vi "RoperGasMeter.vi"() -> ()   [LabVIEW 2012]
uses:
  <vilib>/DAQmx/read.llb/DAQmx Read (Analog 1D DBL NChan 1Samp).vi
  <vilib>/DAQmx/miscellaneous.llb/DAQmx Fill In Error Info.vi
panel:
  out "Meter Flow":string
  out "NG":bool
  out "LP":bool
  out "Meter 6 Present":bool
  out "Meter 5 Present":bool
  out "Meter 4 Present":bool
  out "Meter 3 Present":bool
  out "Meter 2 Present":bool
  out "Meter 1 Present":bool
  out "Meter Type 6":string
  out "Meter Type 2":string
  out "Meter Type 4":string
  out "Meter Type 5":string
  out "Meter Type 3":string
  out "Meter Type 1":string
  out "Meter 6 Size":dbl
  out "Meter 5 Size":dbl
  out "Meter 4 Size":dbl
  out "Meter 3 Size":dbl
  out "Meter 2 Size":dbl
  out "Meter 1 Size":dbl
  out "ANSI Placeholder":dbl
  out "Start Time ANSI":dbl
  in  "Start ANSI":bool
  out "ANSI 5 Minute Average (BTU/hr)":dbl format="%#_5g"
  out "30 Second Average (BTU/hr)":dbl format="%#_5g"
  out "15 Second Average (BTU/hr)":dbl format="%#_5g"
  out "Reference6":dbl
  out "Reference5":dbl
  out "Reference4":dbl
  out "Reference3":dbl
  out "Reference2":dbl
  out "Reference1":dbl
  out "Time":dbl
  out "Num Record":dbl
  in  "HeatingValueLP":dbl=2450.0 min=2400.0 max=2600.0 step=5.0
  out "Output 6":dbl min=0.0 max=5.0 step=0.01
  out "Output 5":dbl min=0.0 max=5.0 step=0.01
  out "Output 4":dbl min=0.0 max=5.0 step=0.01
  out "Output 3":dbl min=0.0 max=5.0 step=0.01
  out "Output 2":dbl min=0.0 max=5.0 step=0.01
  out "Output 1":dbl min=0.0 max=5.0 step=0.01
  out "Signal":bool
  in  "Record":bool
  out "File Path":path
  out "CF/HR":dbl format="%#_2g"
  out "HV":dbl
  in  "HeatingValueNG":dbl=1000.0 min=950.0 max=1150.0 step=1.0
  out "Meter ID":dbl
  out "Gas":string
  out "DisplayChart":cluster{"Flow Rate":dbl}(graph)
  out "Flow Rate":dbl format="%#_5g"
  # "Instant Flow Rate (BTU/hr)"
  # "Dry Heating Value"
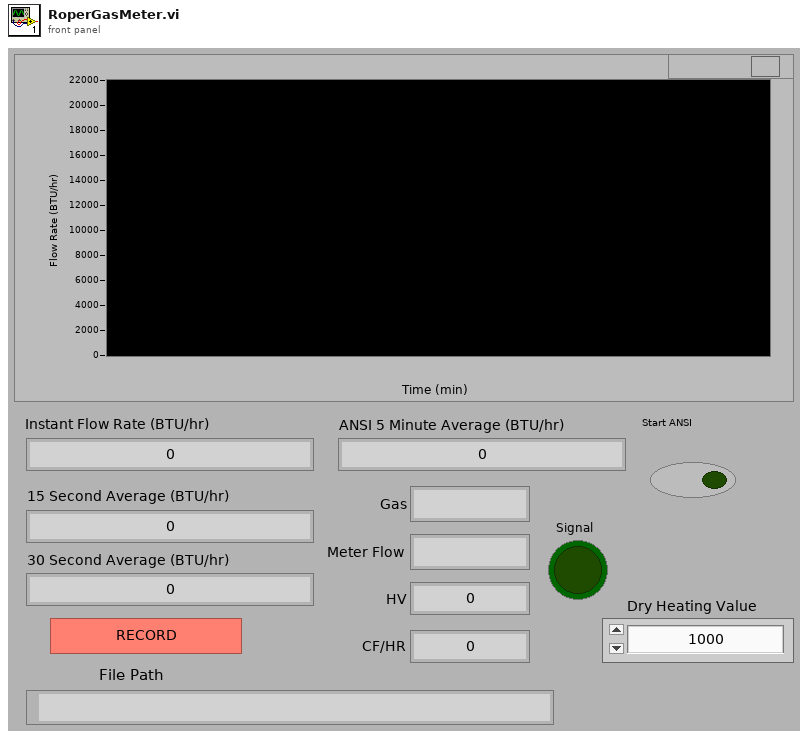
[diagram p1: front panel]
types:
  T1 = enum16{"open", "replace", "create", "open or create", "replace or create", "replace or create with confirmation"}
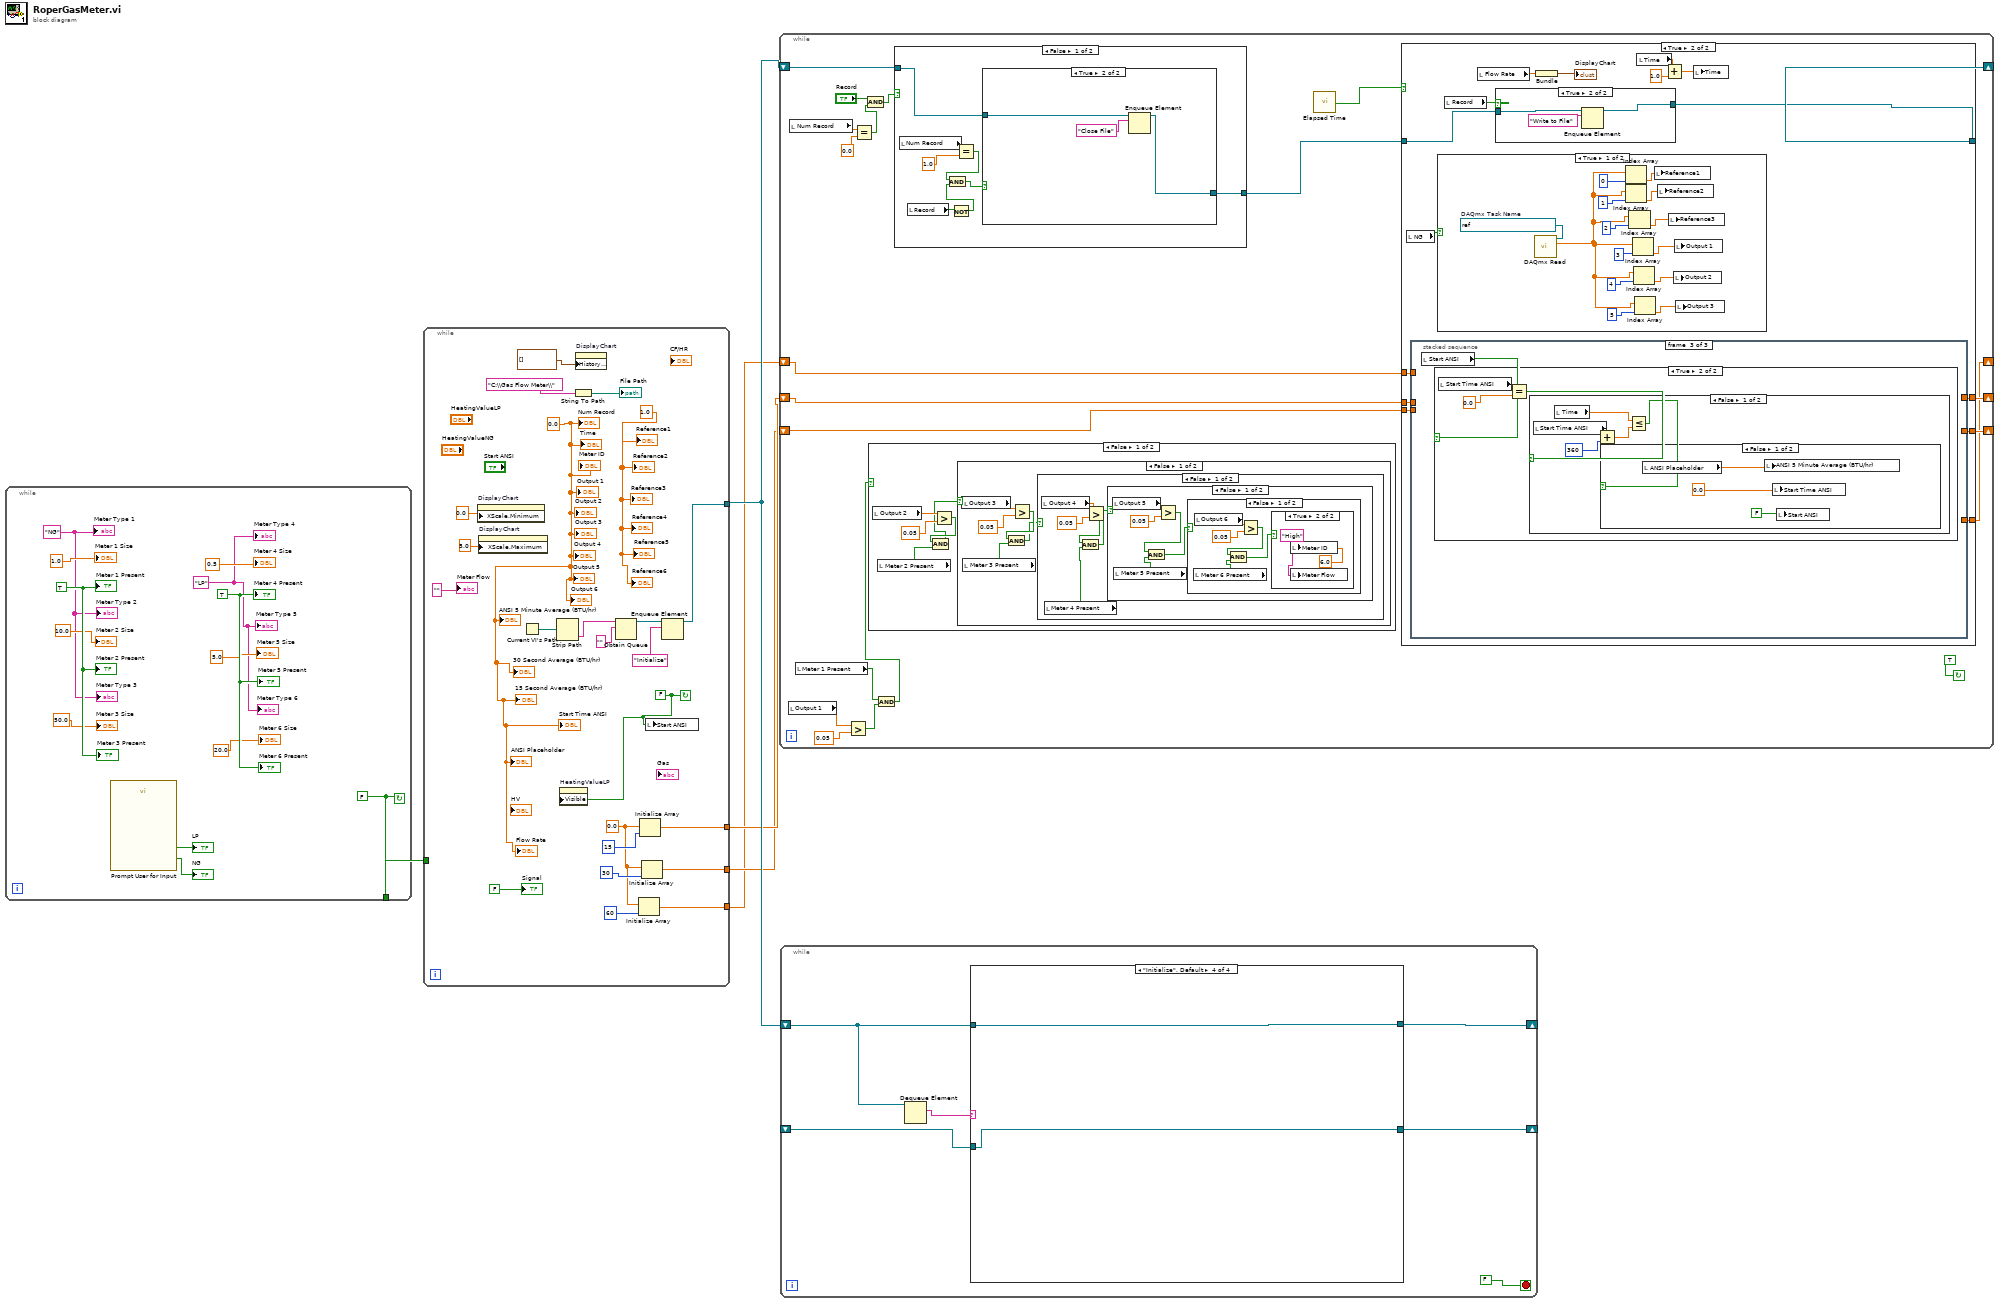
[diagram p0: block diagram]
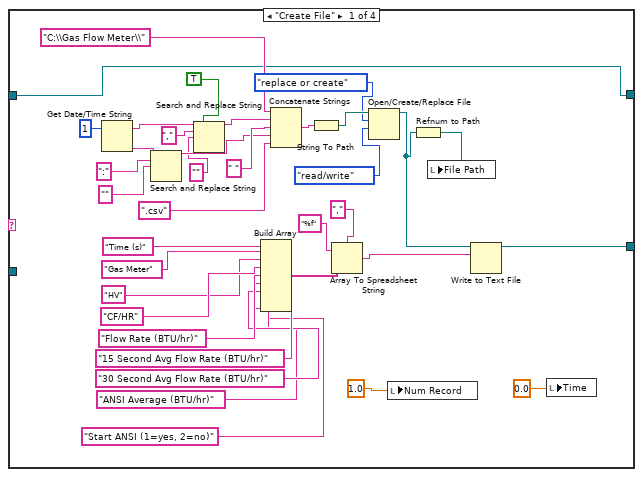
[diagram p2: hidden frame]
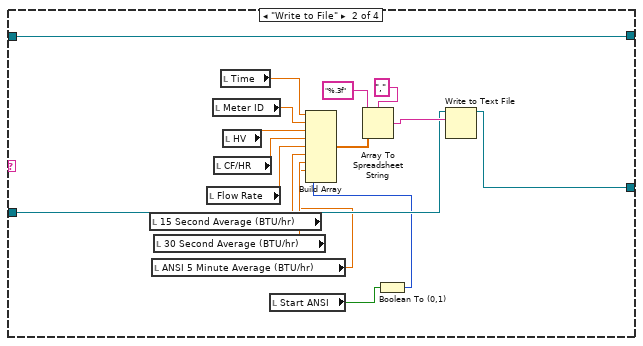
[diagram p3: hidden frame]
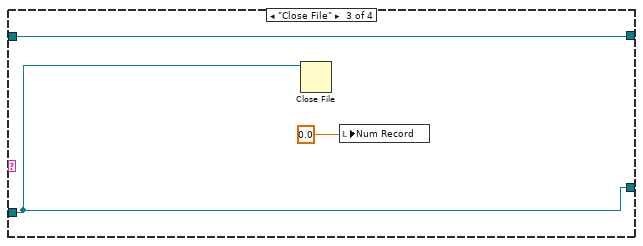
[diagram p4: hidden frame]
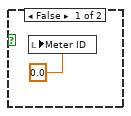
[diagram p5: hidden frame]
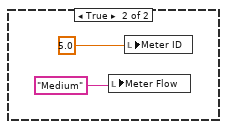
[diagram p6: hidden frame]
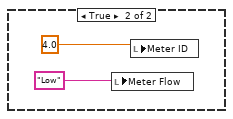
[diagram p7: hidden frame]
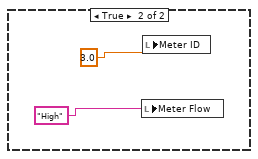
[diagram p8: hidden frame]
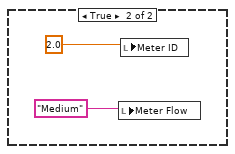
[diagram p9: hidden frame]
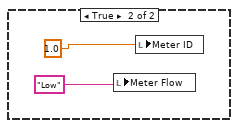
[diagram p10: hidden frame]
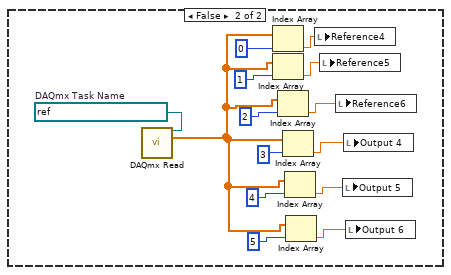
[diagram p12: hidden frame]
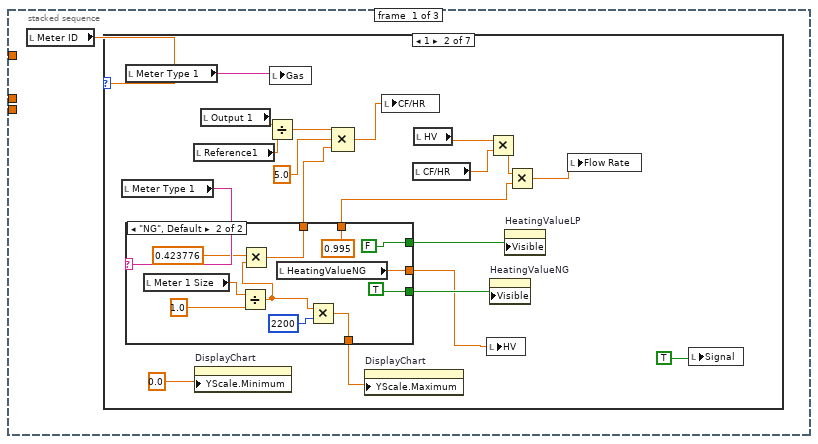
[diagram p13: hidden frame]
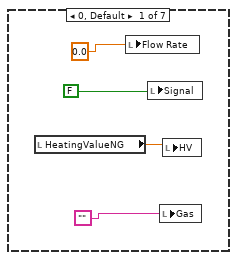
[diagram p14: hidden frame]
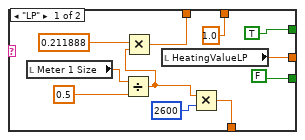
[diagram p15: hidden frame]
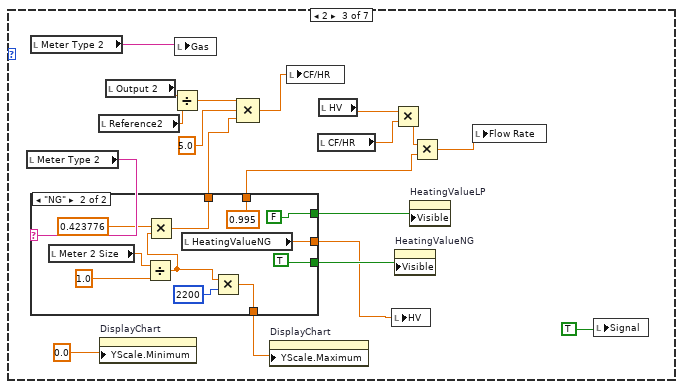
[diagram p16: hidden frame]
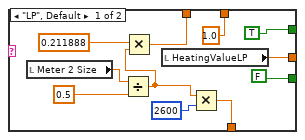
[diagram p17: hidden frame]
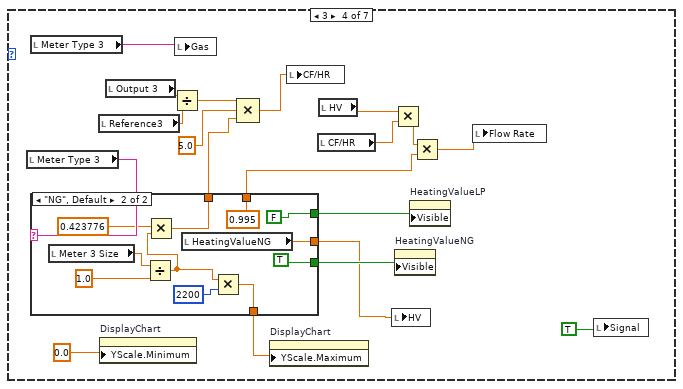
[diagram p18: hidden frame]
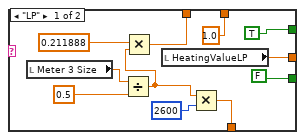
[diagram p19: hidden frame]
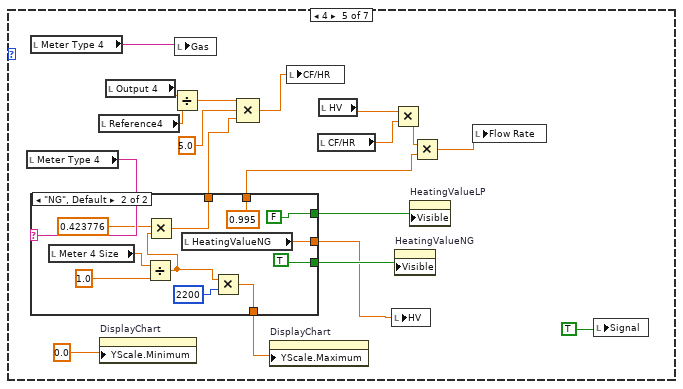
[diagram p20: hidden frame]
diagram:
  n1 = while {
    tunnel: [w18] -> w1
    stop <- w18 continue-if-true
    w6 = "LP"
    w9 = "NG"
    w16 = TRUE
    w17 = TRUE
    w18 = FALSE
    n2 = call "Prompt User for Input"() -> ("NG"=→"NG":bool, "LP"=→"LP":bool)  [unwired: 16 in, 2 out]
    "Meter 4 Size" <- 0.5
    "Meter 5 Size" <- 5.0
    "Meter 2 Size" <- 10.0
    "Meter 1 Size" <- 1.0
    "Meter 6 Size" <- 20.0
    "Meter 3 Size" <- 50.0
    "Meter Type 1" <- w9
    "Meter Type 6" <- w6
    "Meter Type 3" <- w9
    "Meter Type 2" <- w9
    "Meter Type 5" <- w6
    "Meter Type 4" <- w6
    "Meter 1 Present" <- w17
    "Meter 2 Present" <- w17
    "Meter 3 Present" <- w17
    "Meter 4 Present" <- w16
    "Meter 5 Present" <- w16
    "Meter 6 Present" <- w16
  }
  n3 = while {
    tunnel: [w33] -> w5
    tunnel: [w27] -> w4
    tunnel: [w26] -> w3
    tunnel: [w23] -> w2
    tunnel: w1 -> [_]
    stop <- w22 continue-if-true
    w25 = 0.0
    w32 = 1.0
    w21 = 0.0
    w22 = FALSE
    n4 = property on="DisplayChart" class="WFChart (strict)"("XScale.Minimum"=0.0) -> ()  [unwired: 2 in, 2 out]
    n5 = property on="DisplayChart" class="WFChart (strict)"("XScale.Maximum"=5.0) -> ()  [unwired: 2 in, 2 out]
    n6 = Current VI's Path() -> (path=w38:path)
    n7 = Strip Path(path=w38) -> (name=w36:string)  [unwired: 1 out]
    n8 = property on="HeatingValueLP" class="DigNum (strict)"("Visible"=w22) -> ()  [unwired: 2 in, 2 out]
    n9 = String To Path(string="C:\\Gas Flow Meter\\") -> (path=→"File Path":path)
    n10 = property on="DisplayChart" class="WFChart (strict)"("History Data"=cluster{"[0]":dbl}[] []) -> ()  [unwired: 2 in, 2 out]
    n11 = Obtain Queue(name (unnamed)=w36, element data type="") -> (queue out=w34:refnum<queue>)  [unwired: 3 in, 2 out]
    n12 = Initialize Array(w25, 60) -> (w23:dbl[])
    n13 = Initialize Array(w25, 15) -> (w27:dbl[])
    n14 = Initialize Array(w25, 30) -> (w26:dbl[])
    n15 = local write "Start ANSI"(w22) -> ()
    n16 = Enqueue Element(queue=w34, element="Initialize") -> (queue out=w33:refnum<queue>)  [unwired: 2 in, 2 out]
    "Num Record" <- w21
    "Time" <- w21
    "Meter ID" <- w21
    "Output 1" <- w21
    "Output 2" <- w21
    "Output 3" <- w21
    "Output 4" <- w21
    "Output 5" <- w21
    "Output 6" <- w21
    "Reference1" <- w32
    "Reference2" <- w32
    "Reference3" <- w32
    "Reference4" <- w32
    "Reference5" <- w32
    "Reference6" <- w32
    "30 Second Average (BTU/hr)" <- w21
    "15 Second Average (BTU/hr)" <- w21
    "ANSI 5 Minute Average (BTU/hr)" <- w21
    "Start Time ANSI" <- w21
    "ANSI Placeholder" <- w21
    "Flow Rate" <- w21
    "Signal" <- FALSE
    "Meter Flow" <- ""
  }
  n17 = while {
    shift-right: [w54] -> _
    shift-left: w5 -> [w53]
    shift-right: [w50] -> _
    shift-left: w4 -> [w48]
    shift-right: [w49] -> _
    shift-left: w3 -> [w47]
    shift-right: [w46] -> _
    shift-left: w2 -> [w45]
    stop <- TRUE continue-if-true
    n18 = local read "Output 1"() -> (w52:dbl)
    n19 = local read "Num Record"() -> (w58:dbl)
    n20 = local read "Meter 1 Present"() -> (w43:bool)
    n21 = Greater?(x=w52, y=0.05) -> (0:w44:bool)
    n22 = Equal?(x=w58, y=0.0) -> (x = y?=w57:bool)
    n23 = And(x="Record", y=w57) -> (x .and. y?=w56:bool)
    n24 = And(x=w43, y=w44) -> (x .and. y?=w42:bool)
    n25 = case shown="False" w42 {
      frame False {
        n26 = local read "Output 2"() -> (w66:dbl)
        n27 = local read "Meter 2 Present"() -> (w65:bool)
        n28 = Greater?(x=w66, y=0.05) -> (0:w64:bool)
        n29 = And(x=w64, y=w65) -> (x .and. y?=w63:bool)
        n30 = case shown="False" w63 {
          frame False {
            n31 = local read "Output 3"() -> (w71:dbl)
            n32 = local read "Meter 3 Present"() -> (w70:bool)
            n33 = Greater?(x=w71, y=0.05) -> (0:w69:bool)
            n34 = And(x=w69, y=w70) -> (x .and. y?=w68:bool)
            n35 = case shown="False" w68 {
              frame False {
                n36 = local read "Output 4"() -> (w76:dbl)
                n37 = local read "Meter 4 Present"() -> (w75:bool)
                n38 = Greater?(x=w76, y=0.05) -> (0:w74:bool)
                n39 = And(x=w74, y=w75) -> (x .and. y?=w73:bool)
                n40 = case shown="False" w73 {
                  frame False {
                    n41 = local read "Output 5"() -> (w81:dbl)
                    n42 = local read "Meter 5 Present"() -> (w80:bool)
                    n43 = Greater?(x=w81, y=0.05) -> (0:w79:bool)
                    n44 = And(x=w79, y=w80) -> (x .and. y?=w78:bool)
                    n45 = case shown="False" w78 {
                      frame False {
                        n46 = local read "Meter 6 Present"() -> (w85:bool)
                        n47 = local read "Output 6"() -> (w86:dbl)
                        n48 = Greater?(x=w86, y=0.05) -> (0:w84:bool)
                        n49 = And(x=w84, y=w85) -> (x .and. y?=w83:bool)
                        n50 = case shown="True" w83 {
                          frame False {
                            n51 = local write "Meter ID"(0.0) -> ()
                          }
                          frame True {
                            n52 = local write "Meter ID"(6.0) -> ()
                            n53 = local write "Meter Flow"("High") -> ()
                          }
                        }
                      }
                      frame True {
                        n54 = local write "Meter Flow"("Medium") -> ()
                        n55 = local write "Meter ID"(5.0) -> ()
                      }
                    }
                  }
                  frame True {
                    n56 = local write "Meter Flow"("Low") -> ()
                    n57 = local write "Meter ID"(4.0) -> ()
                  }
                }
              }
              frame True {
                n58 = local write "Meter Flow"("High") -> ()
                n59 = local write "Meter ID"(3.0) -> ()
              }
            }
          }
          frame True {
            n60 = local write "Meter Flow"("Medium") -> ()
            n61 = local write "Meter ID"(2.0) -> ()
          }
        }
      }
      frame True {
        n62 = local write "Meter Flow"("Low") -> ()
        n63 = local write "Meter ID"(1.0) -> ()
      }
    }
    n64 = case shown="False" w56 {
      tunnel: w53 -> [w447 w455]
      tunnel: [w446 w454] -> w55
      frame False {
        n65 = local read "Num Record"() -> (w449:dbl)
        n66 = local read "Record"() -> (w443:bool)
        n67 = Not(x=w443) -> (.not. x?=w442:bool)
        n68 = Equal?(x=w449, y=1.0) -> (x = y?=w445:bool)
        n69 = And(x=w445, y=w442) -> (x .and. y?=w444:bool)
        n70 = case shown="True" w444 {
          tunnel: w447 -> [w450 w452]
          tunnel: [w450 w451] -> w446
          frame False {
          }
          frame True {
            n71 = Enqueue Element(queue=w452, element="Close File") -> (queue out=w451:refnum<queue>)  [unwired: 2 in, 2 out]
          }
        }
      }
      frame True {
        n72 = Enqueue Element(queue=w455, element="Create File") -> (queue out=w454:refnum<queue>)  [unwired: 2 in, 2 out]
      }
    }
    n73 = call "Elapsed Time"() -> ("Time has Elapsed"=w61:bool)  [unwired: 12 in, 7 out]
    n74 = case shown="True" w61 {
      tunnel: w55 -> [w104 w113]
      tunnel: [w104 w112] -> w54
      tunnel: w48 -> [w103 w111]
      tunnel: w47 -> [w102 w110]
      tunnel: [w103 w109] -> w50
      tunnel: [w102 w108] -> w49
      tunnel: w45 -> [w101 w107]
      tunnel: [w101 w106] -> w46
      frame False {
      }
      frame True {
        n75 = local read "NG"() -> (w105:bool)
        n76 = stacked-sequence {
          tunnel: w111 -> [_ w423 _]
          tunnel: w110 -> [_ w422 _]
          tunnel: [_ w417 _] -> w109
          tunnel: [_ w413 _] -> w108
          tunnel: w107 -> [_ w407 _]
          tunnel: [_ w404 _] -> w106
          frame #0 {
            n77 = local read "Meter ID"() -> (w148:dbl)
            n78 = case shown="1" w148 {
              frame 0, Default {
                n79 = local read "HeatingValueNG"() -> (w152:dbl)
                n80 = local write "Flow Rate"(0.0) -> ()
                n81 = local write "Signal"(FALSE) -> ()
                n82 = local write "Gas"("") -> ()
                n83 = local write "HV"(w152) -> ()
              }
              frame 1 {
                n84 = local read "Meter Type 1"() -> (w161:string)
                n85 = local read "Meter Type 1"() -> (w155:string)
                n86 = case shown="\"NG\", Default" w161 {
                  tunnel: [w179 w190] -> w160
                  tunnel: [TRUE FALSE] -> w159
                  tunnel: [FALSE TRUE] -> w158
                  tunnel: [1.0 0.995] -> w157
                  tunnel: [w173 w184] -> w156
                  tunnel: [w172 w183] -> w154
                  frame "LP" {
                    n87 = local read "Meter 1 Size"() -> (w181:dbl)
                    n88 = Divide(x=w181, y=0.5) -> (x/y=w174:dbl)
                    n89 = Multiply(x=0.211888, y=w174) -> (x*y=w179:dbl)
                    n90 = local read "HeatingValueLP"() -> (w172:dbl)
                    n91 = Multiply(x=w174, y=2600) -> (x*y=w173:dbl)
                  }
                  frame "NG", Default {
                    n92 = local read "Meter 1 Size"() -> (w192:dbl)
                    n93 = Divide(x=w192, y=1.0) -> (x/y=w185:dbl)
                    n94 = Multiply(x=0.423776, y=w185) -> (x*y=w190:dbl)
                    n95 = local read "HeatingValueNG"() -> (w183:dbl)
                    n96 = Multiply(x=w185, y=2200) -> (x*y=w184:dbl)
                  }
                }
                n97 = local read "Reference1"() -> (w165:dbl)
                n98 = property on="DisplayChart" class="WFChart (strict)"("YScale.Minimum"=0.0) -> ()  [unwired: 2 in, 2 out]
                n99 = local read "Output 1"() -> (w166:dbl)
                n100 = Divide(x=w166, y=w165) -> (x/y=w163:dbl)
                n101 = local write "Gas"(w155) -> ()
                n102 = Compound Arithmetic op=MULTIPLY(w163, 5.0, w160) -> (w153:dbl)
                n103 = property on="DisplayChart" class="WFChart (strict)"("YScale.Maximum"=w156) -> ()  [unwired: 2 in, 2 out]
                n104 = local write "CF/HR"(w153) -> ()
                n105 = local read "CF/HR"() -> (w168:dbl)
                n106 = local read "HV"() -> (w167:dbl)
                n107 = local write "HV"(w154) -> ()
                n108 = Multiply(x=w167, y=w168) -> (x*y=w169:dbl)
                n109 = property on="HeatingValueNG" class="DigNum (strict)"("Visible"=w158) -> ()  [unwired: 2 in, 2 out]
                n110 = property on="HeatingValueLP" class="DigNum (strict)"("Visible"=w159) -> ()  [unwired: 2 in, 2 out]
                n111 = Multiply(x=w169, y=w157) -> (x*y=w170:dbl)
                n112 = local write "Flow Rate"(w170) -> ()
                n113 = local write "Signal"(TRUE) -> ()
              }
              frame 2 {
                n114 = local read "Meter Type 2"() -> (w202:string)
                n115 = local read "Meter Type 2"() -> (w196:string)
                n116 = case shown="\"NG\"" w202 {
                  tunnel: [w220 w231] -> w201
                  tunnel: [TRUE FALSE] -> w200
                  tunnel: [FALSE TRUE] -> w199
                  tunnel: [1.0 0.995] -> w198
                  tunnel: [w214 w225] -> w197
                  tunnel: [w213 w224] -> w195
                  frame "LP", Default {
                    n117 = local read "Meter 2 Size"() -> (w222:dbl)
                    n118 = Divide(x=w222, y=0.5) -> (x/y=w215:dbl)
                    n119 = Multiply(x=0.211888, y=w215) -> (x*y=w220:dbl)
                    n120 = local read "HeatingValueLP"() -> (w213:dbl)
                    n121 = Multiply(x=w215, y=2600) -> (x*y=w214:dbl)
                  }
                  frame "NG" {
                    n122 = local read "Meter 2 Size"() -> (w233:dbl)
                    n123 = Divide(x=w233, y=1.0) -> (x/y=w226:dbl)
                    n124 = Multiply(x=0.423776, y=w226) -> (x*y=w231:dbl)
                    n125 = local read "HeatingValueNG"() -> (w224:dbl)
                    n126 = Multiply(x=w226, y=2200) -> (x*y=w225:dbl)
                  }
                }
                n127 = local read "Reference2"() -> (w206:dbl)
                n128 = property on="DisplayChart" class="WFChart (strict)"("YScale.Minimum"=0.0) -> ()  [unwired: 2 in, 2 out]
                n129 = local read "Output 2"() -> (w207:dbl)
                n130 = Divide(x=w207, y=w206) -> (x/y=w204:dbl)
                n131 = local write "Gas"(w196) -> ()
                n132 = Compound Arithmetic op=MULTIPLY(w204, 5.0, w201) -> (w194:dbl)
                n133 = property on="DisplayChart" class="WFChart (strict)"("YScale.Maximum"=w197) -> ()  [unwired: 2 in, 2 out]
                n134 = local write "CF/HR"(w194) -> ()
                n135 = local read "CF/HR"() -> (w209:dbl)
                n136 = local read "HV"() -> (w208:dbl)
                n137 = local write "HV"(w195) -> ()
                n138 = Multiply(x=w208, y=w209) -> (x*y=w210:dbl)
                n139 = property on="HeatingValueNG" class="DigNum (strict)"("Visible"=w199) -> ()  [unwired: 2 in, 2 out]
                n140 = property on="HeatingValueLP" class="DigNum (strict)"("Visible"=w200) -> ()  [unwired: 2 in, 2 out]
                n141 = Multiply(x=w210, y=w198) -> (x*y=w211:dbl)
                n142 = local write "Flow Rate"(w211) -> ()
                n143 = local write "Signal"(TRUE) -> ()
              }
              frame 3 {
                n144 = local read "Meter Type 3"() -> (w243:string)
                n145 = local read "Meter Type 3"() -> (w237:string)
                n146 = case shown="\"NG\", Default" w243 {
                  tunnel: [w261 w272] -> w242
                  tunnel: [TRUE FALSE] -> w241
                  tunnel: [FALSE TRUE] -> w240
                  tunnel: [1.0 0.995] -> w239
                  tunnel: [w255 w266] -> w238
                  tunnel: [w254 w265] -> w236
                  frame "LP" {
                    n147 = local read "Meter 3 Size"() -> (w263:dbl)
                    n148 = Divide(x=w263, y=0.5) -> (x/y=w256:dbl)
                    n149 = Multiply(x=0.211888, y=w256) -> (x*y=w261:dbl)
                    n150 = local read "HeatingValueLP"() -> (w254:dbl)
                    n151 = Multiply(x=w256, y=2600) -> (x*y=w255:dbl)
                  }
                  frame "NG", Default {
                    n152 = local read "Meter 3 Size"() -> (w274:dbl)
                    n153 = Divide(x=w274, y=1.0) -> (x/y=w267:dbl)
                    n154 = Multiply(x=0.423776, y=w267) -> (x*y=w272:dbl)
                    n155 = local read "HeatingValueNG"() -> (w265:dbl)
                    n156 = Multiply(x=w267, y=2200) -> (x*y=w266:dbl)
                  }
                }
                n157 = local read "Reference3"() -> (w247:dbl)
                n158 = property on="DisplayChart" class="WFChart (strict)"("YScale.Minimum"=0.0) -> ()  [unwired: 2 in, 2 out]
                n159 = local read "Output 3"() -> (w248:dbl)
                n160 = Divide(x=w248, y=w247) -> (x/y=w245:dbl)
                n161 = local write "Gas"(w237) -> ()
                n162 = Compound Arithmetic op=MULTIPLY(w245, 5.0, w242) -> (w235:dbl)
                n163 = property on="DisplayChart" class="WFChart (strict)"("YScale.Maximum"=w238) -> ()  [unwired: 2 in, 2 out]
                n164 = local write "CF/HR"(w235) -> ()
                n165 = local read "CF/HR"() -> (w250:dbl)
                n166 = local read "HV"() -> (w249:dbl)
                n167 = local write "HV"(w236) -> ()
                n168 = Multiply(x=w249, y=w250) -> (x*y=w251:dbl)
                n169 = property on="HeatingValueNG" class="DigNum (strict)"("Visible"=w240) -> ()  [unwired: 2 in, 2 out]
                n170 = property on="HeatingValueLP" class="DigNum (strict)"("Visible"=w241) -> ()  [unwired: 2 in, 2 out]
                n171 = Multiply(x=w251, y=w239) -> (x*y=w252:dbl)
                n172 = local write "Flow Rate"(w252) -> ()
                n173 = local write "Signal"(TRUE) -> ()
              }
              frame 4 {
                n174 = local read "Meter Type 4"() -> (w284:string)
                n175 = local read "Meter Type 4"() -> (w278:string)
                n176 = case shown="\"NG\", Default" w284 {
                  tunnel: [w302 w313] -> w283
                  tunnel: [TRUE FALSE] -> w282
                  tunnel: [FALSE TRUE] -> w281
                  tunnel: [1.0 0.995] -> w280
                  tunnel: [w296 w307] -> w279
                  tunnel: [w295 w306] -> w277
                  frame "LP" {
                    n177 = local read "Meter 4 Size"() -> (w304:dbl)
                    n178 = Divide(x=w304, y=0.5) -> (x/y=w297:dbl)
                    n179 = Multiply(x=0.211888, y=w297) -> (x*y=w302:dbl)
                    n180 = local read "HeatingValueLP"() -> (w295:dbl)
                    n181 = Multiply(x=w297, y=2600) -> (x*y=w296:dbl)
                  }
                  frame "NG", Default {
                    n182 = local read "Meter 4 Size"() -> (w315:dbl)
                    n183 = Divide(x=w315, y=1.0) -> (x/y=w308:dbl)
                    n184 = Multiply(x=0.423776, y=w308) -> (x*y=w313:dbl)
                    n185 = local read "HeatingValueNG"() -> (w306:dbl)
                    n186 = Multiply(x=w308, y=2200) -> (x*y=w307:dbl)
                  }
                }
                n187 = local read "Reference4"() -> (w288:dbl)
                n188 = property on="DisplayChart" class="WFChart (strict)"("YScale.Minimum"=0.0) -> ()  [unwired: 2 in, 2 out]
                n189 = local read "Output 4"() -> (w289:dbl)
                n190 = Divide(x=w289, y=w288) -> (x/y=w286:dbl)
                n191 = local write "Gas"(w278) -> ()
                n192 = Compound Arithmetic op=MULTIPLY(w286, 5.0, w283) -> (w276:dbl)
                n193 = property on="DisplayChart" class="WFChart (strict)"("YScale.Maximum"=w279) -> ()  [unwired: 2 in, 2 out]
                n194 = local write "CF/HR"(w276) -> ()
                n195 = local read "CF/HR"() -> (w291:dbl)
                n196 = local read "HV"() -> (w290:dbl)
                n197 = local write "HV"(w277) -> ()
                n198 = Multiply(x=w290, y=w291) -> (x*y=w292:dbl)
                n199 = property on="HeatingValueNG" class="DigNum (strict)"("Visible"=w281) -> ()  [unwired: 2 in, 2 out]
                n200 = property on="HeatingValueLP" class="DigNum (strict)"("Visible"=w282) -> ()  [unwired: 2 in, 2 out]
                n201 = Multiply(x=w292, y=w280) -> (x*y=w293:dbl)
                n202 = local write "Flow Rate"(w293) -> ()
                n203 = local write "Signal"(TRUE) -> ()
              }
              frame 5 {
                n204 = local read "Meter Type 5"() -> (w325:string)
                n205 = local read "Meter Type 5"() -> (w319:string)
                n206 = case shown="\"NG\", Default" w325 {
                  tunnel: [w343 w354] -> w324
                  tunnel: [TRUE FALSE] -> w323
                  tunnel: [FALSE TRUE] -> w322
                  tunnel: [1.0 0.995] -> w321
                  tunnel: [w337 w348] -> w320
                  tunnel: [w336 w347] -> w318
                  frame "LP" {
                    n207 = local read "Meter 5 Size"() -> (w345:dbl)
                    n208 = Divide(x=w345, y=0.5) -> (x/y=w338:dbl)
                    n209 = Multiply(x=0.211888, y=w338) -> (x*y=w343:dbl)
                    n210 = local read "HeatingValueLP"() -> (w336:dbl)
                    n211 = Multiply(x=w338, y=2600) -> (x*y=w337:dbl)
                  }
                  frame "NG", Default {
                    n212 = local read "Meter 5 Size"() -> (w356:dbl)
                    n213 = Divide(x=w356, y=1.0) -> (x/y=w349:dbl)
                    n214 = Multiply(x=0.423776, y=w349) -> (x*y=w354:dbl)
                    n215 = local read "HeatingValueNG"() -> (w347:dbl)
                    n216 = Multiply(x=w349, y=2200) -> (x*y=w348:dbl)
                  }
                }
                n217 = local read "Reference5"() -> (w329:dbl)
                n218 = property on="DisplayChart" class="WFChart (strict)"("YScale.Minimum"=0.0) -> ()  [unwired: 2 in, 2 out]
                n219 = local read "Output 5"() -> (w330:dbl)
                n220 = Divide(x=w330, y=w329) -> (x/y=w327:dbl)
                n221 = local write "Gas"(w319) -> ()
                n222 = Compound Arithmetic op=MULTIPLY(w327, 5.0, w324) -> (w317:dbl)
                n223 = property on="DisplayChart" class="WFChart (strict)"("YScale.Maximum"=w320) -> ()  [unwired: 2 in, 2 out]
                n224 = local write "CF/HR"(w317) -> ()
                n225 = local read "CF/HR"() -> (w332:dbl)
                n226 = local read "HV"() -> (w331:dbl)
                n227 = local write "HV"(w318) -> ()
                n228 = Multiply(x=w331, y=w332) -> (x*y=w333:dbl)
                n229 = property on="HeatingValueNG" class="DigNum (strict)"("Visible"=w322) -> ()  [unwired: 2 in, 2 out]
                n230 = property on="HeatingValueLP" class="DigNum (strict)"("Visible"=w323) -> ()  [unwired: 2 in, 2 out]
                n231 = Multiply(x=w333, y=w321) -> (x*y=w334:dbl)
                n232 = local write "Flow Rate"(w334) -> ()
                n233 = local write "Signal"(TRUE) -> ()
              }
              frame 6 {
                n234 = local read "Meter Type 6"() -> (w366:string)
                n235 = local read "Meter Type 6"() -> (w360:string)
                n236 = case shown="\"NG\", Default" w366 {
                  tunnel: [w384 w395] -> w365
                  tunnel: [TRUE FALSE] -> w364
                  tunnel: [FALSE TRUE] -> w363
                  tunnel: [1.0 0.995] -> w362
                  tunnel: [w378 w389] -> w361
                  tunnel: [w377 w388] -> w359
                  frame "LP" {
                    n237 = local read "Meter 6 Size"() -> (w386:dbl)
                    n238 = Divide(x=w386, y=0.5) -> (x/y=w379:dbl)
                    n239 = Multiply(x=0.211888, y=w379) -> (x*y=w384:dbl)
                    n240 = local read "HeatingValueLP"() -> (w377:dbl)
                    n241 = Multiply(x=w379, y=2600) -> (x*y=w378:dbl)
                  }
                  frame "NG", Default {
                    n242 = local read "Meter 6 Size"() -> (w397:dbl)
                    n243 = Divide(x=w397, y=1.0) -> (x/y=w390:dbl)
                    n244 = Multiply(x=0.423776, y=w390) -> (x*y=w395:dbl)
                    n245 = local read "HeatingValueNG"() -> (w388:dbl)
                    n246 = Multiply(x=w390, y=2200) -> (x*y=w389:dbl)
                  }
                }
                n247 = local read "Reference6"() -> (w370:dbl)
                n248 = property on="DisplayChart" class="WFChart (strict)"("YScale.Minimum"=0.0) -> ()  [unwired: 2 in, 2 out]
                n249 = local read "Output 6"() -> (w371:dbl)
                n250 = Divide(x=w371, y=w370) -> (x/y=w368:dbl)
                n251 = local write "Gas"(w360) -> ()
                n252 = Compound Arithmetic op=MULTIPLY(w368, 5.0, w365) -> (w358:dbl)
                n253 = property on="DisplayChart" class="WFChart (strict)"("YScale.Maximum"=w361) -> ()  [unwired: 2 in, 2 out]
                n254 = local write "CF/HR"(w358) -> ()
                n255 = local read "CF/HR"() -> (w373:dbl)
                n256 = local read "HV"() -> (w372:dbl)
                n257 = local write "HV"(w359) -> ()
                n258 = Multiply(x=w372, y=w373) -> (x*y=w374:dbl)
                n259 = property on="HeatingValueNG" class="DigNum (strict)"("Visible"=w363) -> ()  [unwired: 2 in, 2 out]
                n260 = property on="HeatingValueLP" class="DigNum (strict)"("Visible"=w364) -> ()  [unwired: 2 in, 2 out]
                n261 = Multiply(x=w374, y=w362) -> (x*y=w375:dbl)
                n262 = local write "Flow Rate"(w375) -> ()
                n263 = local write "Signal"(TRUE) -> ()
              }
            }
          }
          frame #1 {
            n264 = Delete From Array(array=w423, index=14) -> (array with subset deleted=w418:dbl[])  [unwired: 1 in, 1 out]
            n265 = Delete From Array(array=w407, index=59) -> (array with subset deleted=w405:dbl[])  [unwired: 1 in, 1 out]
            n266 = Delete From Array(array=w422, index=29) -> (array with subset deleted=w419:dbl[])  [unwired: 1 in, 1 out]
            n267 = local read "Flow Rate"() -> (w400:dbl)
            n268 = Insert Into Array(array=w405, index=0, new element=w400) -> (w404:dbl[])
            n269 = Insert Into Array(array=w418, index=0, new element=w400) -> (w417:dbl[])
            n270 = Insert Into Array(array=w419, index=0, new element=w400) -> (w413:dbl[])
            n271 = Add Array Elements(numeric array=w404) -> (sum=w403:dbl)
            n272 = Array Size(array=w404) -> (size(s)=w402:i32)
            n273 = Add Array Elements(numeric array=w413) -> (sum=w412:dbl)
            n274 = Array Size(array=w413) -> (size(s)=w411:i32)
            n275 = Add Array Elements(numeric array=w417) -> (sum=w415:dbl)
            n276 = Array Size(array=w417) -> (size(s)=w416:i32)
            n277 = Divide(x=w403, y=w402) -> (x/y=w401:dbl)
            n278 = Divide(x=w412, y=w411) -> (x/y=w410:dbl)
            n279 = Divide(x=w415, y=w416) -> (x/y=w414:dbl)
            n280 = local write "15 Second Average (BTU/hr)"(w414) -> ()
            n281 = local write "ANSI Placeholder"(w401) -> ()
            n282 = local write "30 Second Average (BTU/hr)"(w410) -> ()
          }
          frame #2 {
            n283 = local read "Start ANSI"() -> (w424:bool)
            n284 = case shown="True" w424 {
              frame False {
              }
              frame True {
                n285 = local read "Start Time ANSI"() -> (w426:dbl)
                n286 = Equal?(x=w426, y=0.0) -> (x = y?=w425:bool)
                n287 = case shown="False" w425 {
                  frame False {
                    n288 = local read "Start Time ANSI"() -> (w432:dbl)
                    n289 = local read "Time"() -> (w429:dbl)
                    n290 = Add(x=w432, y=360) -> (x+y=w430:dbl)
                    n291 = Less Or Equal?(x=w429, y=w430) -> (x <= y?=w428:bool)
                    n292 = case shown="False" w428 {
                      frame False {
                        n293 = local read "ANSI Placeholder"() -> (w434:dbl)
                        n294 = local write "ANSI 5 Minute Average (BTU/hr)"(w434) -> ()
                        n295 = local write "Start Time ANSI"(0.0) -> ()
                        n296 = local write "Start ANSI"(FALSE) -> ()
                      }
                      frame True {
                      }
                    }
                  }
                  frame True {
                    n297 = local read "Time"() -> (w437:dbl)
                    n298 = local write "ANSI 5 Minute Average (BTU/hr)"(0.0) -> ()
                    n299 = local write "Start Time ANSI"(w437) -> ()
                  }
                }
              }
            }
          }
        }
        n300 = case shown="True" w105 {
          frame True {
            w133 = refnum<k21> "ReadNGFlowMeterIn"  # DAQmx Task Name
            n301 = call-poly <vilib>:"DAQmx Read.vi"("task/channels in"=w133) -> ("data"=w124:dbl[])  [unwired: 12 in, 2 out]
            n302 = Index Array(array=w124, index=0) -> (element=w129:dbl)
            n303 = Index Array(array=w124, index=1) -> (element=w130:dbl)
            n304 = Index Array(array=w124, index=2) -> (element=w123:dbl)
            n305 = Index Array(array=w124, index=3) -> (element=w122:dbl)
            n306 = Index Array(array=w124, index=4) -> (element=w121:dbl)
            n307 = Index Array(array=w124, index=5) -> (element=w120:dbl)
            n308 = local write "Reference1"(w129) -> ()
            n309 = local write "Reference2"(w130) -> ()
            n310 = local write "Reference3"(w123) -> ()
            n311 = local write "Output 2"(w121) -> ()
            n312 = local write "Output 1"(w122) -> ()
            n313 = local write "Output 3"(w120) -> ()
          }
          frame False {
            w147 = refnum<k21> "ReadLPFlowMeterIn"  # DAQmx Task Name
            n314 = call-poly <vilib>:"DAQmx Read.vi"("task/channels in"=w147) -> ("data"=w138:dbl[])  [unwired: 12 in, 2 out]
            n315 = Index Array(array=w138, index=0) -> (element=w143:dbl)
            n316 = Index Array(array=w138, index=1) -> (element=w144:dbl)
            n317 = Index Array(array=w138, index=2) -> (element=w137:dbl)
            n318 = Index Array(array=w138, index=3) -> (element=w136:dbl)
            n319 = Index Array(array=w138, index=4) -> (element=w135:dbl)
            n320 = Index Array(array=w138, index=5) -> (element=w134:dbl)
            n321 = local write "Reference4"(w143) -> ()
            n322 = local write "Reference5"(w144) -> ()
            n323 = local write "Reference6"(w137) -> ()
            n324 = local write "Output 5"(w135) -> ()
            n325 = local write "Output 4"(w136) -> ()
            n326 = local write "Output 6"(w134) -> ()
          }
        }
        n327 = local read "Record"() -> (w117:bool)
        n328 = local read "Flow Rate"() -> (w119:dbl)
        n329 = case shown="True" w117 {
          tunnel: w113 -> [w438 w440]
          tunnel: [w438 w439] -> w112
          frame False {
          }
          frame True {
            n330 = Enqueue Element(queue=w440, element="Write to File") -> (queue out=w439:refnum<queue>)  [unwired: 2 in, 2 out]
          }
        }
        n331 = Bundle("Flow Rate"=w119) -> (→"DisplayChart":cluster{"Flow Rate":dbl})  [unwired: 1 in]
        n332 = local read "Time"() -> (w115:dbl)
        n333 = Add(x=w115, y=1.0) -> (x+y=w114:dbl)
        n334 = local write "Time"(w114) -> ()
      }
    }
  }
  n335 = while {
    shift-right: [w460] -> _
    shift-left: w5 -> [w457]
    shift-right: [w459] -> _
    shift-left: _ -> [w458]
    stop <- FALSE stop-if-true
    n336 = Dequeue Element(queue=w457) -> (element=w461:string)  [unwired: 2 in, 3 out]
    n337 = case shown="\"Initialize\", Default" w461 {
      tunnel: [w468 w506 w517 w520] -> w460
      tunnel: w457 -> [w468 w506 w517 w520]
      tunnel: [w467 w504 w516 w519] -> w459
      tunnel: w458 -> [_ w505 w516 w519]
      frame "Create File" {
        n338 = Get Date/Time String(date format (0)=1) -> (date string=w473:string, time string=w470:string)  [unwired: 2 in]
        n339 = Search and Replace String(input string=w470, search string=":", replace string="") -> (result string=w479:string)  [unwired: 5 in, 3 out]
        n340 = Search and Replace String(replace all?=TRUE, input string=w473, search string=",", replace string="") -> (result string=w480:string)  [unwired: 4 in, 3 out]
        n341 = Build Array("Time (s)", "Gas Meter", "HV", "CF/HR", "Flow Rate (BTU/hr)", "15 Second Avg Flow Rate (BTU/hr)", "30 Second Avg Flow Rate (BTU/hr)", "ANSI Average (BTU/hr)", "Start ANSI (1=yes, 2=no)") -> (w490:string[])
        n342 = Concatenate Strings("C:\\Gas Flow Meter\\", w480, " ", w479, ".csv") -> (w476:string)
        n343 = String To Path(string=w476) -> (path=w496:path)
        n344 = Array To Spreadsheet String(delimiter (Tab)=",", array=w490, 3:"%f" ("format string")) -> (spreadsheet string=w491:string)
        n345 = Open/Create/Replace File(file path (use dialog)=w496, operation (0:open)=T1."replace or create", access (0:read/write)=enum16{"read/write", "read-only", "write-only"}."read/write") -> (refnum out=w498:refnum<file>)  [unwired: 3 in, 2 out]
        n346 = local write "Num Record"(1.0) -> ()
        n347 = Refnum to Path(1:w498) -> (0:w497:path)
        n348 = local write "File Path"(w497) -> ()
        n349 = Write to Text File(file (use dialog)=w498, text=w491) -> (refnum out=w467:refnum<file>)  [unwired: 2 in, 2 out]
        n350 = local write "Time"(0.0) -> ()
      }
      frame "Write to File" {
        n351 = local read "15 Second Average (BTU/hr)"() -> (w502:dbl)
        n352 = local read "ANSI 5 Minute Average (BTU/hr)"() -> (w501:dbl)
        n353 = local read "30 Second Average (BTU/hr)"() -> (w503:dbl)
        n354 = local read "Flow Rate"() -> (w509:dbl)
        n355 = local read "Meter ID"() -> (w512:dbl)
        n356 = local read "CF/HR"() -> (w510:dbl)
        n357 = local read "Time"() -> (w513:dbl)
        n358 = local read "HV"() -> (w511:dbl)
        n359 = local read "Start ANSI"() -> (w500:bool)
        n360 = Boolean To (0,1)(Boolean=w500) -> (0, 1=w499:i16)
        n361 = Build Array(w513, w512, w511, w510, w509, w502, w503, w501, w499) -> (w508:dbl[])
        n362 = Array To Spreadsheet String(delimiter (Tab)=",", array=w508, 3:"%.3f" ("format string")) -> (spreadsheet string=w507:string)
        n363 = Write to Text File(file (use dialog)=w505, text=w507) -> (refnum out=w504:refnum<file>)  [unwired: 2 in, 2 out]
      }
      frame "Close File" {
        n364 = Close File(refnum=w516) -> ()  [unwired: 1 in, 2 out]
        n365 = local write "Num Record"(0.0) -> ()
      }
      frame "Initialize", Default {
      }
    }
  }
